vi "BracePLUS_Serial_Interface.vi"(10 "Serial Settings":T2={"baud rate"=115200, "data bits"=8, "parity"=enum."None", "stop bits"=10, "flow control"=0} {"flow control" items=["None"=0, "XON/XOFF"=1, "RTS/CTS"=2, "DTR/DSR"=4]; "stop bits" items=["1.0"=10, "1.5"=15, "2.0"=20]; "data bits" min=5 max=8 step=1; "baud rate" items=["75"=75, "110"=110, "134"=134, "150"=150, "300"=300, "600"=600, "1200"=1200, "1800"=1800, "2400"=2400, "4800"=4800, "7200"=7200, "9600"=9600, "14400"=14400, "19200"=19200, "28800"=28800, "38400"=38400, "56000"=56000, "57600"=57600, "115200"=115200, "128000"=128000, "230400"=230400]}, 11 "VISA Resource\nName":refnum<visa-resource-name>="COM3") -> ()   [LabVIEW 2018]
uses:
  <vilib>/Math Plots/3D Math Plots/3D Surface/3D Surface XCtrl/3D Surface.xctl
panel:
  in  "Tab Control":T1(tab)
  in  "Connect Button":bool
  out "Connected":bool
  out "Initialised":bool
  in  "Visualize?":bool
  in  "Stream":bool
  in  "Stop stream":bool
  out "3D Surface":refnum<class "3D Plot Datatype.lvclass">[](xcontrol)
  out "Logging to file:":string
  in  "Open Data Folder":bool
  in  "Open Button":bool
  out "filenames":string[](array[string])
  out "Initialisation String":string
  out "Data Packet":string
  out "Packets in":i32
  out "Data Path":path
  out "Real dT":u32
  out "Reading":bool
  out "Time (s)":dbl format="%.2f"
  in  "Packet Size (Bytes)":u32=128
  in  "dT":u32=40
  in  "Tare?":bool
  out "B xyz":dbl[][](array[numeric])
  out "Average Y":dbl format="%0.2f"
  out "Average X":dbl format="%0.2f"
  out "Node Position":dbl[][](array[numeric])
  in  "stop":bool
  # "Brace+ Interface"
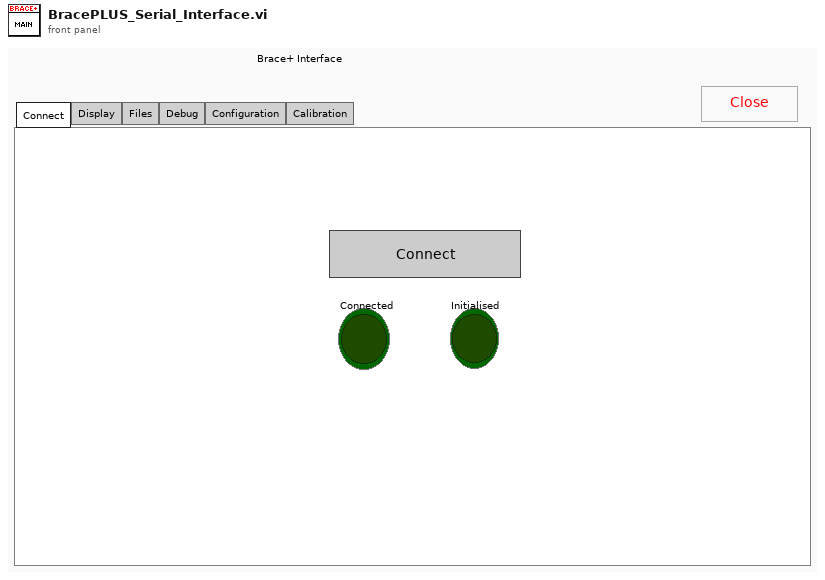
[diagram p1: front panel]
types:
  T1 = enum32{"Connect", "Display", "Files", "Debug", "Configuration", "Calibration"}
  T2 = cluster{"baud rate":u32, "data bits":u16, "parity":enum16{"None", "Odd", "Even", "Mark", "Space"}, "stop bits":u16, "flow control":u16}
  T3 = enum16{"big-endian, network order", "native, host order", "little-endian"}
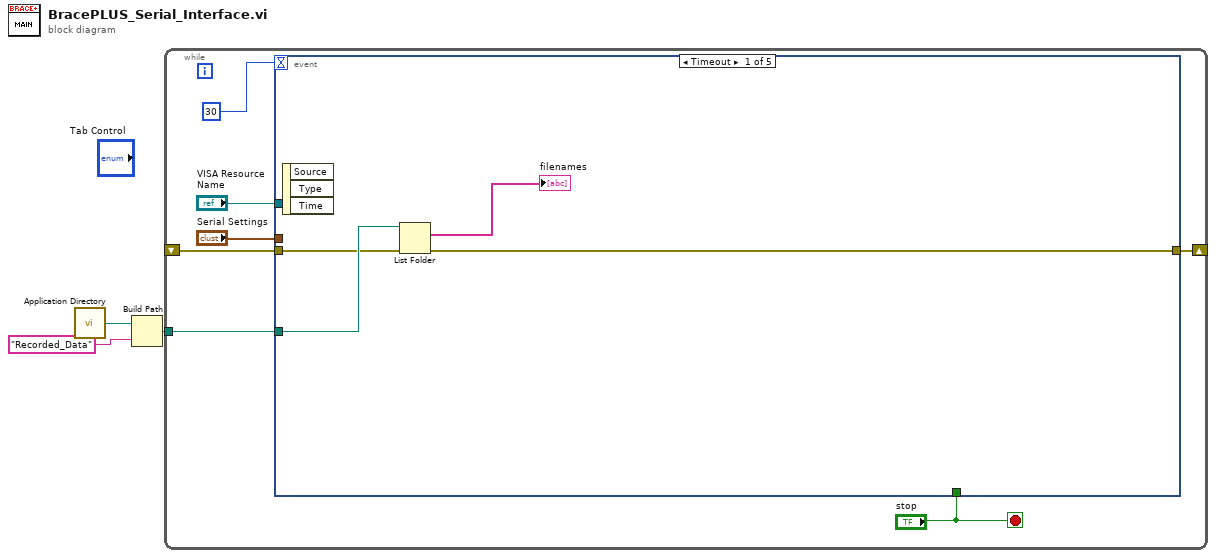
[diagram p0: block diagram]
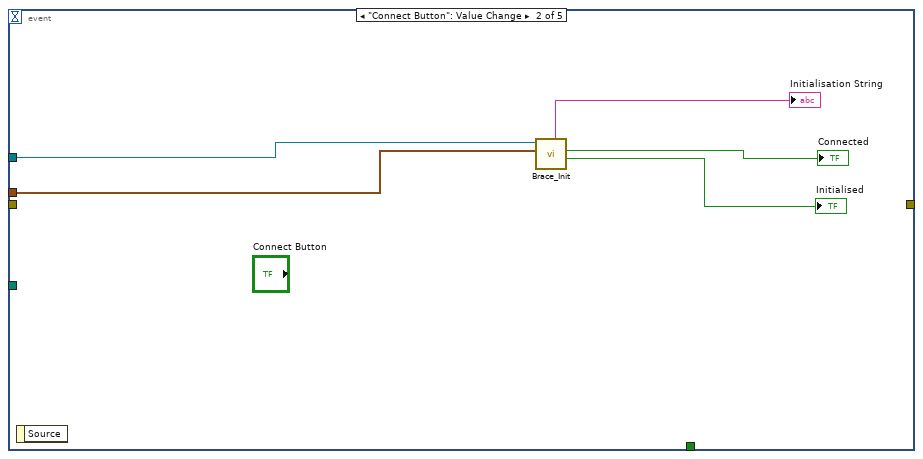
[diagram p2: hidden frame]
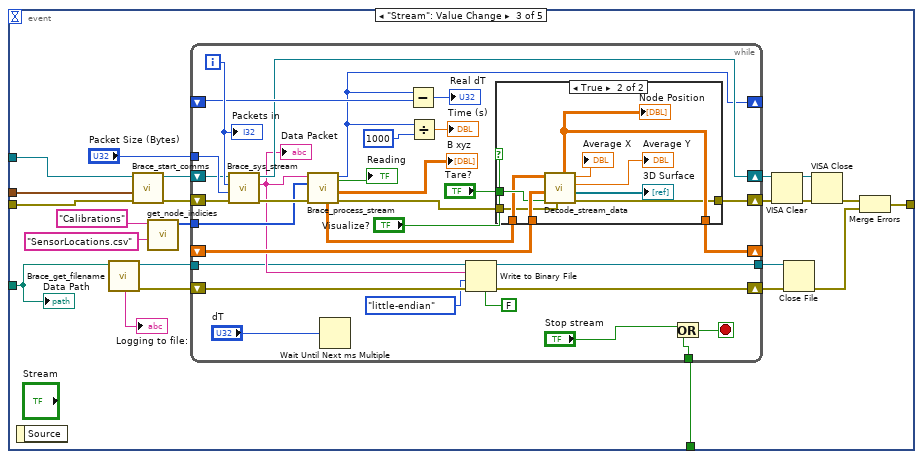
[diagram p3: hidden frame]
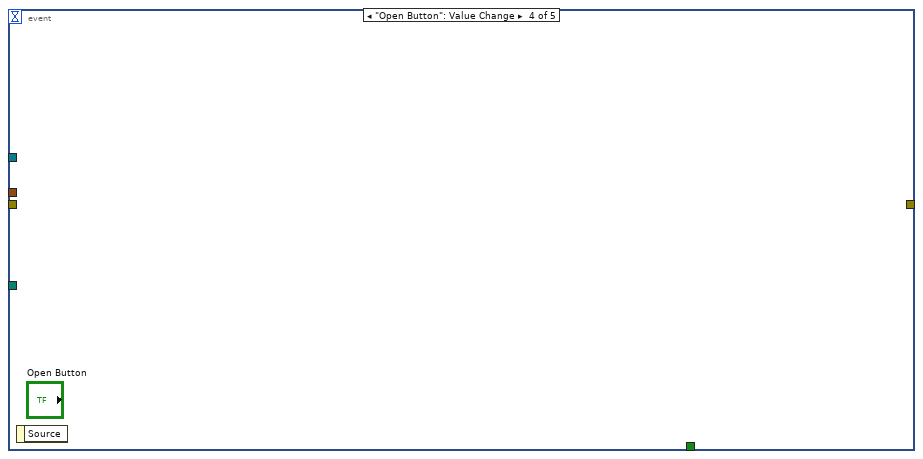
[diagram p5: hidden frame]
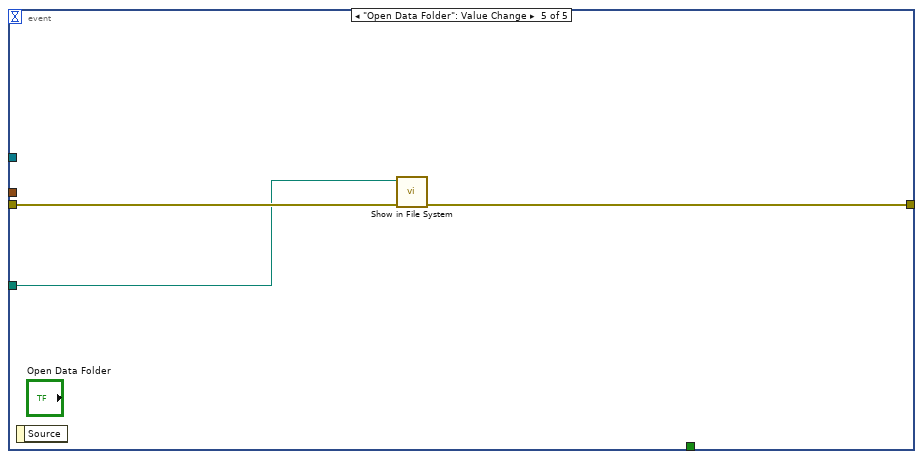
[diagram p6: hidden frame]
diagram:
  n1 = call <vilib>:"Application Directory.vi"() -> ("Application Directory"=w2:path)
  n2 = Build Path(base path=w2, name or relative path="Recorded_Data" ("string")) -> (appended path=w1:path)
  n3 = while {
    shift-right: [w6] -> _
    shift-left: _ -> [w10]
    tunnel: w1 -> [w5]
    stop <- "stop" stop-if-true
    n4 = event shown="[0] Timeout" {
      selector: _ -> [_ _ _ _ _]
      dyn-events: _ -> [_ _ _ _ _]
      timeout: 30 -> [_ _ _ _ _]
      tunnel: w10 -> [w13 _ w34 _ w87]
      tunnel: "Serial Settings" -> [_ w19 w33 _ _]
      tunnel: "VISA Resource\nName" -> [_ w18 w32 _ _]
      tunnel: [w11 _ w25 _ w88] -> w6
      tunnel: w5 -> [w14 _ w22 _ w86]
      tunnel: "stop" -> [_ _ w20 _ _]
      event Timeout {
        n5 = event-data() -> ()  [unwired: 1 in, 3 out]
        n6 = List Folder(path=w14, error in=w13) -> (filenames=→"filenames":string[], error out=w11:errorcluster)  [unwired: 2 in, 2 out]
      }
      event "Connect Button": Value Change {
        n7 = event-data() -> ()  [unwired: 1 in, 1 out]
        n8 = call "Brace_Init.vi"("Serial Settings"=w19, "VISA Refnum in"=w18) -> ("Initialised"=→"Initialised":bool, "Connected"=→"Connected":bool, "Data Out"=→"Initialisation String":string)  [unwired: 7 in]
      }
      event "Stream": Value Change {
        n9 = event-data() -> ()  [unwired: 1 in, 1 out]
        n10 = call "Brace_get_filename.vi"("Directory"=w22) -> ("error out"=w24:errorcluster, "Filename"=→"Logging to file:":string, "refnum out"=w23:refnum<file>)  [unwired: 8 in]
        n11 = call "Brace_start_comms.vi"("error in (no error)"=w34, "Serial Settings"=w33, "VISA resource name"=w32) -> ("error out"=w35:errorcluster, "VISA Refnum out"=w31:refnum<visa-resource-name>)  [unwired: 7 in]
        n12 = call "get_node_indicies.vi"("File"="SensorLocations.csv", "Calibrations"="Calibrations") -> ("Sensor Indicies"=w37:i32[])  [unwired: 9 in]
        n13 = while {
          shift-right: [w70] -> _
          shift-left: _ -> [w71]
          shift-right: [w64] -> _
          shift-left: _ -> [w67]
          tunnel: w37 -> [w69]
          tunnel: "Packet Size (Bytes)" -> [w68]
          shift-right: [w65] -> w30
          shift-left: w31 -> [w66]
          shift-right: [w43] -> w42
          shift-left: w35 -> [w72]
          shift-right: [w58] -> w29
          shift-left: w24 -> [w60]
          tunnel: [w57] -> w28
          tunnel: w23 -> [w47]
          tunnel: w20 -> [w45]
          i -> [w73]
          stop <- w46 stop-if-true
          n14 = call "Brace_sys_stream.vi"("error in (no error)"=w72, "Packet Size (Bytes)"=w68, "Numeric"=w73, "VISA Refnum in"=w66) -> ("error out"=w74:errorcluster, "Data Out"=w61:string, "VISA Refnum out"=w65:refnum<visa-resource-name>)  [unwired: 5 in]
          "Data Packet" <- w61
          n15 = call "Brace_process_stream.vi"("error in (no error)"=w74, "Sensor Indicies"=w69, "Data Packet"=w61) -> ("error out"=w44:errorcluster, "B xyz"=→"B xyz":dbl[][], "Time out"=w64:u32, "Sensors (uT)"=w53:dbl[][], "Boolean"=→"Reading":bool)  [unwired: 4 in]
          n16 = Wait Until Next ms Multiple(millisecond multiple="dT") -> ()  [unwired: 1 out]
          n17 = Subtract(x=w64, y=w67) -> (x-y=→"Real dT":u32)
          n18 = Divide(x=w64, y=u32 1000) -> (x/y=→"Time (s)":dbl)
          n19 = Write to Binary File(file (use dialog)=w47, data=w61, error in=w60, 5:FALSE ("prepend array or string size? (T)"), 9:T3."little-endian" ("byte order (0:big-endian, network order)")) -> (refnum out=w57:refnum<file>, error out=w58:errorcluster)  [unwired: 1 in, 1 out]
          n20 = case shown="True" "Visualize?" {
            tunnel: w71 -> [_ w85]
            tunnel: [w76 w84] -> w70
            tunnel: "Tare?" -> [_ w83]
            tunnel: w53 -> [w76 w79]
            tunnel: w44 -> [w75 w78]
            tunnel: [w75 w77] -> w43
            frame False {
            }
            frame True {
              n21 = call "Decode_stream_data.vi"("Error In"=w78, "Tare"=w83, "Sensor Output - Position (mm) 2"=w85, "Bxyz"=w79) -> ("Error Out"=w77:errorcluster, "3D Plot lvclass Array out"=→"3D Surface":refnum<class "3D Plot Datatype.lvclass">[], "mean 2"=→"Average Y":dbl, "mean"=→"Average X":dbl, "Sensor Output - Position (mm) 3"=w84:dbl[][])  [unwired: 3 in]
              "Node Position" <- w84
            }
          }
          n22 = Or(x="Stop stream", y=w45) -> (x .or. y?=w46:bool)
          "Packets in" <- w73
        }
        n23 = VISA Clear(VISA resource name=w30, error in (no error)=w42) -> (VISA resource name out=w41:refnum<visa-resource-name>, error out=w40:errorcluster)
        n24 = Close File(refnum=w28, error in=w29) -> (error out=w26:errorcluster)  [unwired: 1 out]
        n25 = VISA Close(VISA resource name=w41, error in (no error)=w40) -> (error out=w27:errorcluster)
        n26 = Merge Errors(w27, w26) -> (w25:errorcluster)
        "Data Path" <- w22
      }
      event "Open Button": Value Change {
        n27 = event-data() -> ()  [unwired: 1 in, 1 out]
      }
      event "Open Data Folder": Value Change {
        n28 = event-data() -> ()  [unwired: 1 in, 1 out]
        n29 = call <vilib>:"Show in File System.vi"("error in (no error)"=w87, "file or directory path"=w86) -> ("error out"=w88:errorcluster)  [unwired: 9 in]
      }
    }
  }
